vi "Serial.vi"() -> ()   [LabVIEW 2016]
uses:
  <vilib>/Instr/_visa.llb/VISA Configure Serial Port (Instr).vi
panel:
  in  "byte count":u32
  in  "stop":bool
  in  "VISA resource name":refnum<visa-resource-name>
  out "read buffer":string
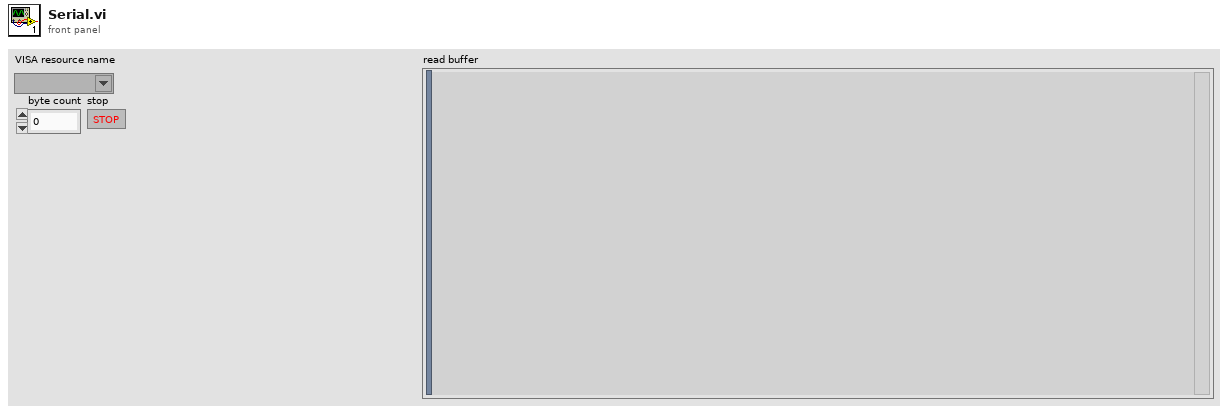
[diagram p1: front panel]
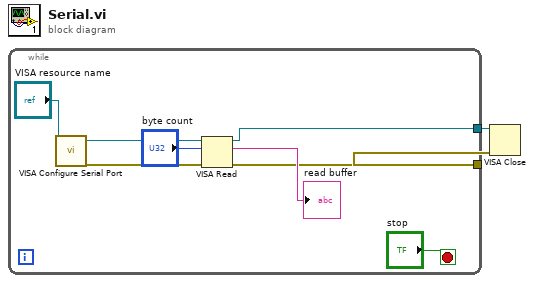
[diagram p0: block diagram]
diagram:
  n1 = while {
    tunnel: [w6] -> w2
    tunnel: [w5] -> w1
    stop <- "stop" stop-if-true
    n2 = call-poly "VISA Configure Serial Port"("VISA resource name"="VISA resource name") -> ("VISA resource name out"=w10:refnum<visa-resource-name>, "error out"=w9:errorcluster)  [unwired: 13 in]
    n3 = VISA Read(VISA resource name=w10, byte count="byte count", error in (no error)=w9) -> (VISA resource name out=w6:refnum<visa-resource-name>, read buffer=→"read buffer":string, error out=w5:errorcluster)  [unwired: 1 out]
  }
  n4 = VISA Close(VISA resource name=w2, error in (no error)=w1) -> ()  [unwired: 1 out]
